vi "DMSO_load_sample_BM.vi"(6 "COM Port":refnum<visa-resource-name>="COM9", 7 "Pump Parameters":T1={"Speed 1"="100", "Speed 2"="250", "Speed 3"="250", "Speed 4"="250", "UW/Sample"="5", "Sparge"="2", "Std"="4", "Waste"="15", "Air"="14", "Milli-Q"="1", "H2SO4"="6", "NaOH"="3", "Catalyst"="7", "Cell (H+ side)"="8", "Cell (sample side)"="9", "NaCl"="9"}, 9 "step to ml":dbl=1920.0, 10 "Total Vol. (mL)":dbl, 11 "Sample Vol. (mL)":dbl=10.0) -> ()   [LabVIEW 2021]
panel:
  out "Full Command":string="o4A0V5000o1P14400o4D14400o1P33600o4D9600o2D24000o5P9600o2D9600o6P33600o4D33600"
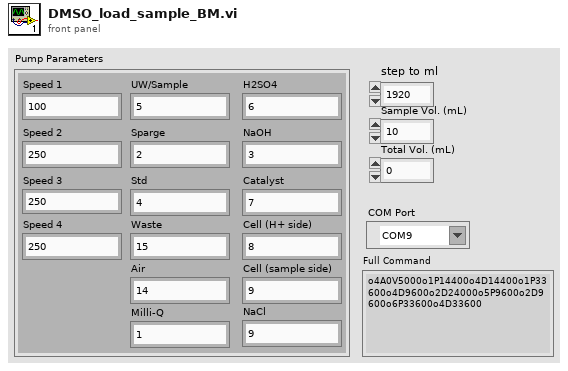
[diagram p1: front panel]
types:
  T1 = cluster{"Speed 1":string, "Speed 2":string, "Speed 3":string, "Speed 4":string, "UW/Sample":string, "Sparge":string, "Std":string, "Waste":string, "Air":string, "Milli-Q":string, "H2SO4":string, "NaOH":string, "Catalyst":string, "Cell (H+ side)":string, "Cell (sample side)":string, "NaCl":string}
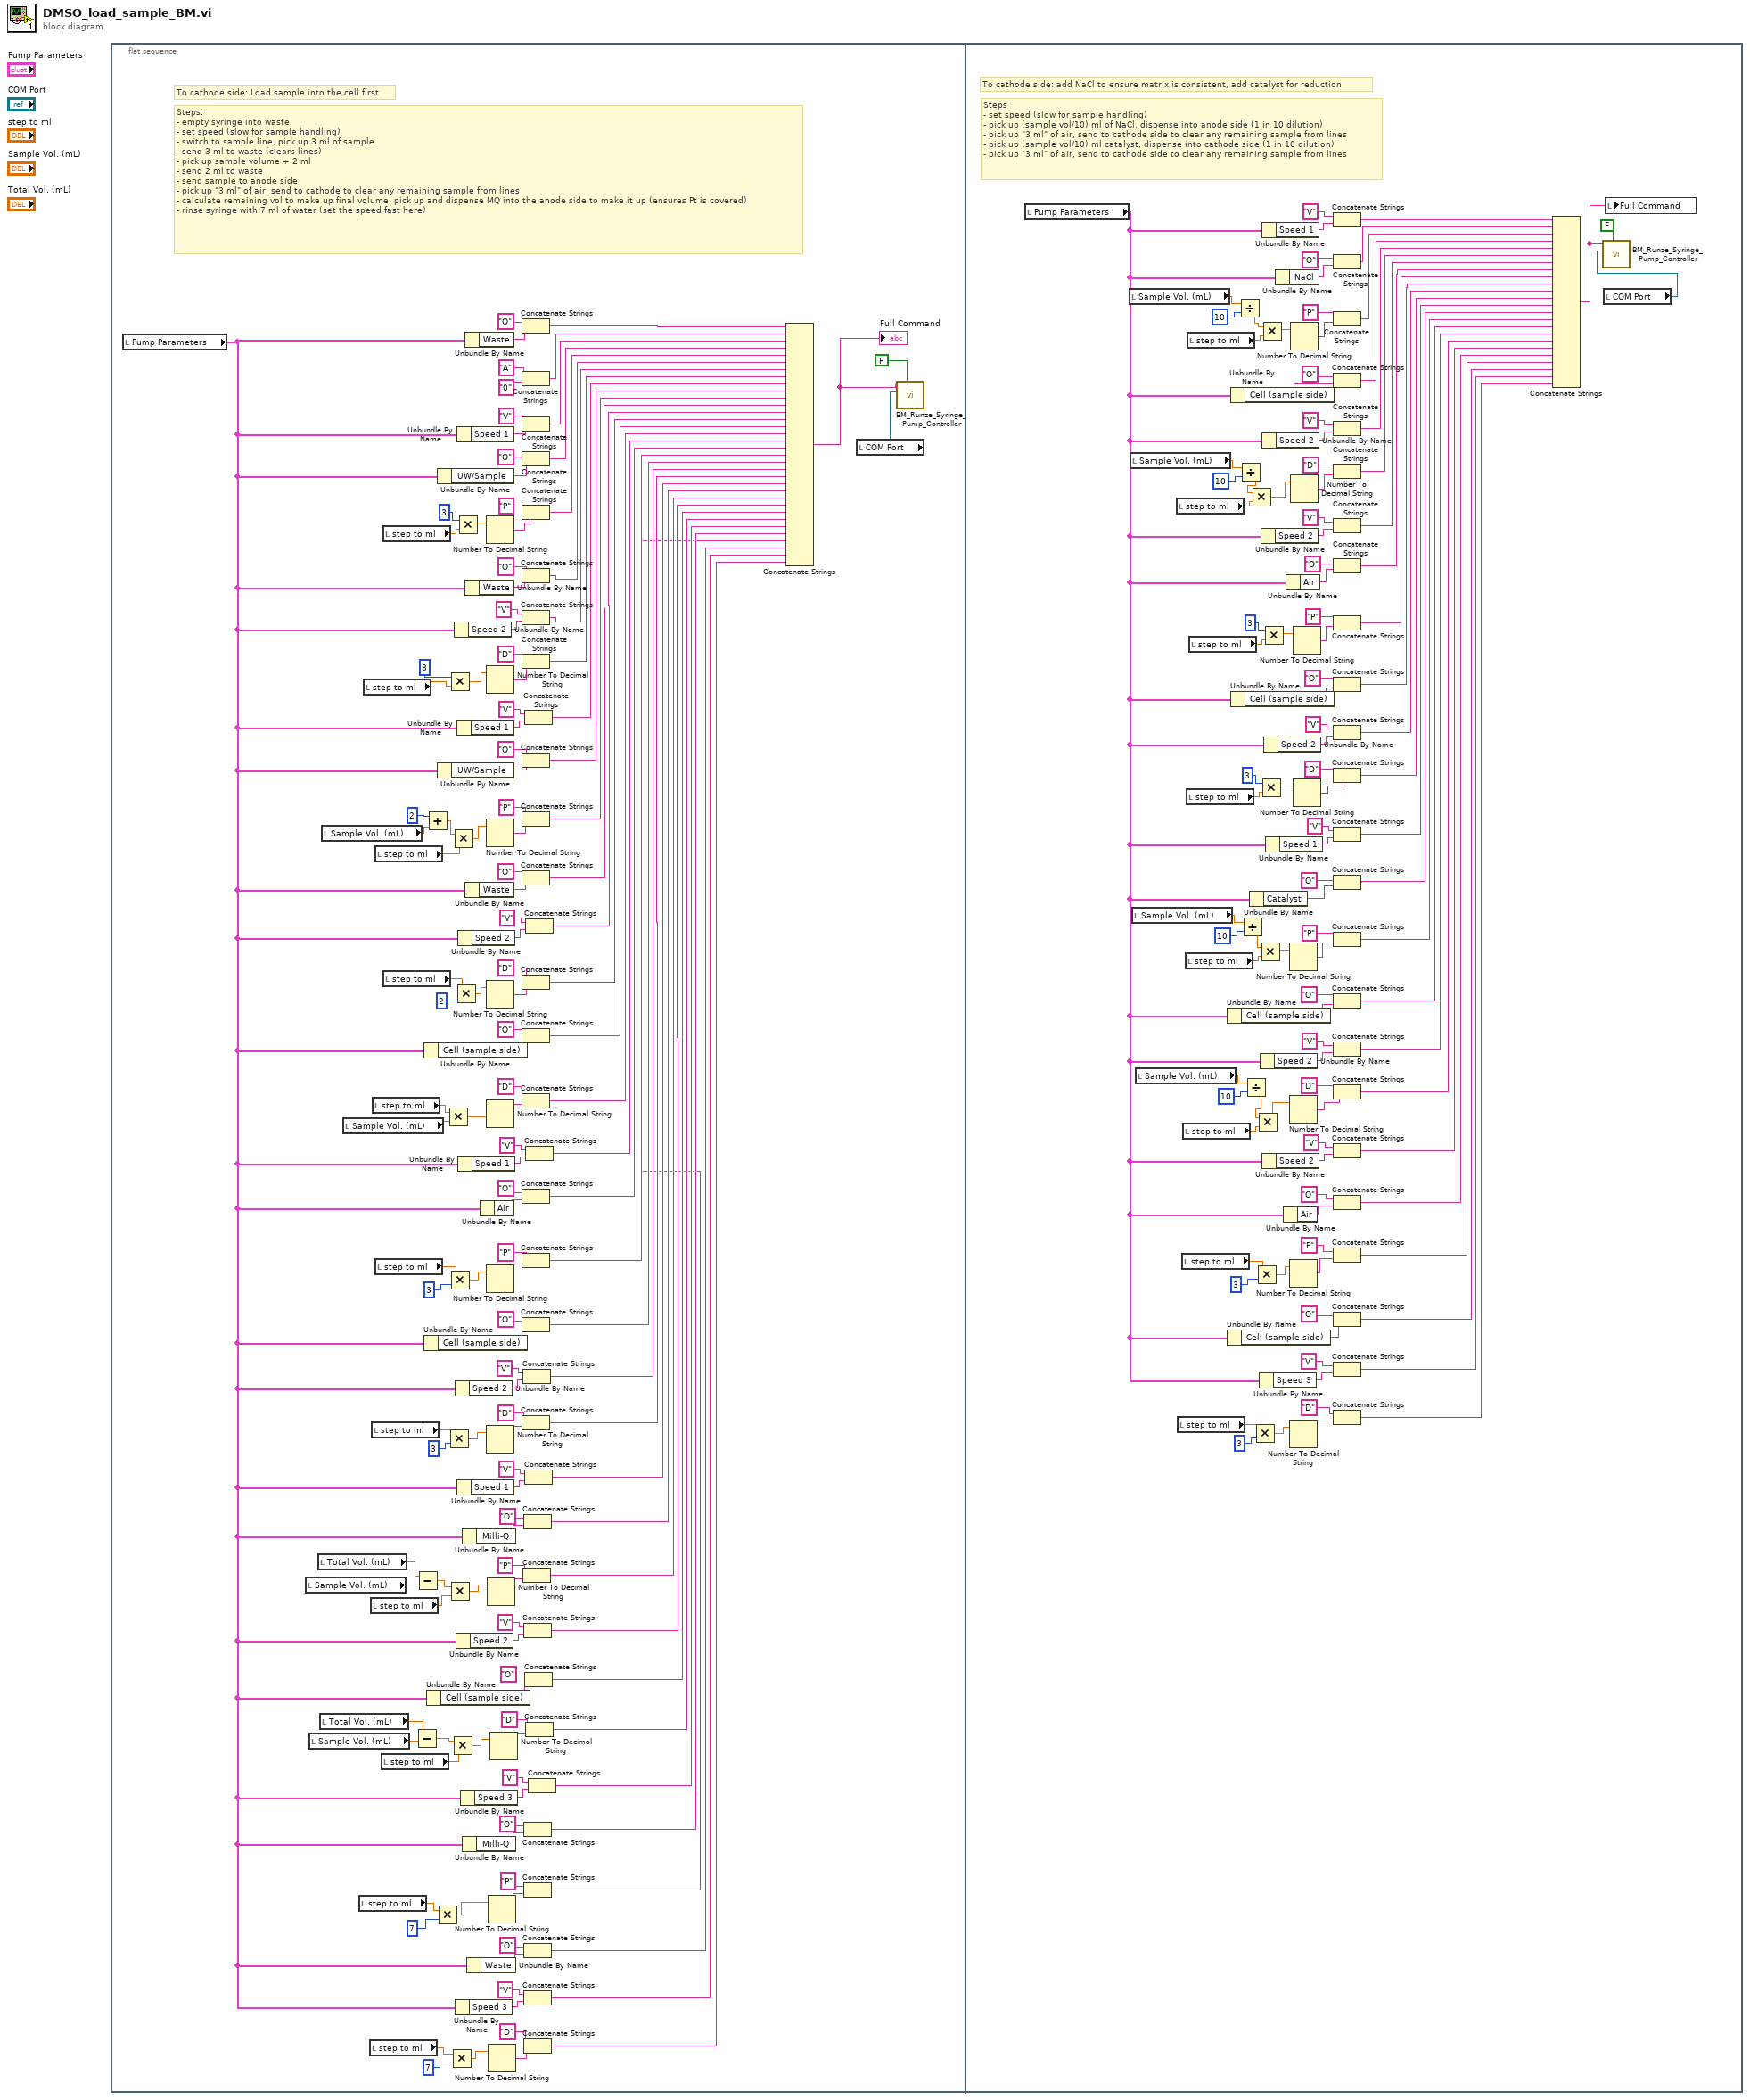
[diagram p0: block diagram]
diagram:
  n1 = flat-sequence {
    frame #0 {
      # "Steps:\n- empty syringe into waste\n- set speed (slow for sample handling)\n- switch to sample line, pick up 3 ml of sample\n- send 3 ml to waste (clears lines)\n- pick up sample volume + 2 ml\n- send 2 ml to waste\n- send sample to anode side\n- pick up \"3 ml\" of air, send to cathode to clear any remaining sample from lines\n- calculate remaining vol to make up final volume; pick up and dispense MQ into the anode side to make it up (ensures Pt is covered)\n- rinse syringe with 7 ml of water (set the speed fast here)"
      # "To cathode side: Load sample into the cell first"
      n2 = local read "Pump Parameters"() -> (w3:T1)
      n3 = local read "Sample Vol. (mL)"() -> (w2:dbl)
      n4 = local read "Sample Vol. (mL)"() -> (w1:dbl)
      n5 = local read "Total Vol. (mL)"() -> (w23:dbl)
      n6 = local read "Total Vol. (mL)"() -> (w22:dbl)
      n7 = local read "Sample Vol. (mL)"() -> (w103:dbl)
      n8 = local read "Sample Vol. (mL)"() -> (w102:dbl)
      n9 = local read "step to ml"() -> (w115:dbl)
      n10 = local read "step to ml"() -> (w97:dbl)
      n11 = local read "step to ml"() -> (w77:dbl)
      n12 = local read "step to ml"() -> (w29:dbl)
      n13 = local read "step to ml"() -> (w86:dbl)
      n14 = local read "step to ml"() -> (w117:dbl)
      n15 = local read "step to ml"() -> (w118:dbl)
      n16 = local read "step to ml"() -> (w116:dbl)
      n17 = local read "step to ml"() -> (w20:dbl)
      n18 = local read "step to ml"() -> (w120:dbl)
      n19 = local read "step to ml"() -> (w119:dbl)
      n20 = Subtract(x=w22, y=w1) -> (x-y=w21:dbl)
      n21 = Subtract(x=w23, y=w2) -> (x-y=w30:dbl)
      n22 = Add(x=2, y=w103) -> (x+y=w138:dbl)
      n23 = Unbundle By Name(w3) -> ("Cell (sample side)"=w108:string)
      n24 = Unbundle By Name(w3) -> ("Cell (sample side)"=w106:string)
      n25 = Unbundle By Name(w3) -> ("Cell (sample side)"=w27:string)
      n26 = Multiply(x=w115, y=7) -> (x*y=w135:dbl)
      n27 = Unbundle By Name(w3) -> ("UW/Sample"=w112:string)
      n28 = Unbundle By Name(w3) -> ("UW/Sample"=w110:string)
      n29 = Multiply(x=w117, y=w102) -> (x*y=w142:dbl)
      n30 = Multiply(x=w86, y=3) -> (x*y=w87:dbl)
      n31 = Multiply(x=3, y=w97) -> (x*y=w98:dbl)
      n32 = Multiply(x=w116, y=3) -> (x*y=w141:dbl)
      n33 = Multiply(x=w30, y=w29) -> (x*y=w33:dbl)
      n34 = Multiply(x=w77, y=7) -> (x*y=w79:dbl)
      n35 = Multiply(x=w21, y=w20) -> (x*y=w26:dbl)
      n36 = Multiply(x=w138, y=w118) -> (x*y=w139:dbl)
      n37 = Multiply(x=w119, y=2) -> (x*y=w144:dbl)
      n38 = Multiply(x=3, y=w120) -> (x*y=w136:dbl)
      n39 = Unbundle By Name(w3) -> ("Speed 2"=w72:string)
      n40 = Unbundle By Name(w3) -> ("Speed 2"=w64:string)
      n41 = Unbundle By Name(w3) -> ("Speed 3"=w15:string)
      n42 = Unbundle By Name(w3) -> ("Speed 2"=w18:string)
      n43 = Unbundle By Name(w3) -> ("Speed 1"=w113:string)
      n44 = Unbundle By Name(w3) -> ("Speed 1"=w71:string)
      n45 = Unbundle By Name(w3) -> ("Speed 1"=w63:string)
      n46 = Unbundle By Name(w3) -> ("Speed 2"=w68:string)
      n47 = Unbundle By Name(w3) -> ("Speed 1"=w67:string)
      n48 = Unbundle By Name(w3) -> ("Speed 3"=w17:string)
      n49 = Unbundle By Name(w3) -> ("Milli-Q"=w34:string)
      n50 = Unbundle By Name(w3) -> ("Milli-Q"=w105:string)
      n51 = Unbundle By Name(w3) -> ("Waste"=w114:string)
      n52 = Unbundle By Name(w3) -> ("Waste"=w111:string)
      n53 = Unbundle By Name(w3) -> ("Waste"=w109:string)
      n54 = Unbundle By Name(w3) -> ("Waste"=w104:string)
      n55 = Unbundle By Name(w3) -> ("Air"=w107:string)
      n56 = Number To Decimal String(number=w136) -> (decimal integer string=w96:string)  [unwired: 1 out]
      n57 = Number To Decimal String(number=w98) -> (decimal integer string=w95:string)  [unwired: 1 out]
      n58 = Number To Decimal String(number=w139) -> (decimal integer string=w93:string)  [unwired: 1 out]
      n59 = Number To Decimal String(number=w144) -> (decimal integer string=w92:string)  [unwired: 1 out]
      n60 = Number To Decimal String(number=w142) -> (decimal integer string=w89:string)  [unwired: 1 out]
      n61 = Number To Decimal String(number=w141) -> (decimal integer string=w84:string)  [unwired: 1 out]
      n62 = Number To Decimal String(number=w87) -> (decimal integer string=w82:string)  [unwired: 1 out]
      n63 = Number To Decimal String(number=w33) -> (decimal integer string=w31:string)  [unwired: 1 out]
      n64 = Number To Decimal String(number=w135) -> (decimal integer string=w80:string)  [unwired: 1 out]
      n65 = Number To Decimal String(number=w79) -> (decimal integer string=w76:string)  [unwired: 1 out]
      n66 = Number To Decimal String(number=w26) -> (decimal integer string=w24:string)  [unwired: 1 out]
      n67 = Concatenate Strings("O", w114) -> (w59:string)
      n68 = Concatenate Strings("A", "0") -> (w58:string)
      n69 = Concatenate Strings("V", w113) -> (w57:string)
      n70 = Concatenate Strings("O", w112) -> (w56:string)
      n71 = Concatenate Strings("P", w96) -> (w55:string)
      n72 = Concatenate Strings("O", w111) -> (w54:string)
      n73 = Concatenate Strings("V", w72) -> (w53:string)
      n74 = Concatenate Strings("D", w95) -> (w52:string)
      n75 = Concatenate Strings("O", w110) -> (w50:string)
      n76 = Concatenate Strings("P", w93) -> (w49:string)
      n77 = Concatenate Strings("O", w109) -> (w48:string)
      n78 = Concatenate Strings("D", w92) -> (w46:string)
      n79 = Concatenate Strings("O", w108) -> (w45:string)
      n80 = Concatenate Strings("D", w89) -> (w44:string)
      n81 = Concatenate Strings("O", w107) -> (w42:string)
      n82 = Concatenate Strings("P", w84) -> (w41:string)
      n83 = Concatenate Strings("O", w106) -> (w40:string)
      n84 = Concatenate Strings("D", w82) -> (w38:string)
      n85 = Concatenate Strings("V", w64) -> (w39:string)
      n86 = Concatenate Strings("P", w31) -> (w13:string)
      n87 = Concatenate Strings("O", w34) -> (w14:string)
      n88 = Concatenate Strings("V", w18) -> (w12:string)
      n89 = Concatenate Strings("O", w105) -> (w8:string)
      n90 = Concatenate Strings("P", w80) -> (w7:string)
      n91 = Concatenate Strings("O", w104) -> (w6:string)
      n92 = Concatenate Strings("V", w15) -> (w5:string)
      n93 = Concatenate Strings("D", w76) -> (w4:string)
      n94 = Concatenate Strings("V", w71) -> (w51:string)
      n95 = Concatenate Strings("V", w63) -> (w37:string)
      n96 = Concatenate Strings("O", w27) -> (w11:string)
      n97 = Concatenate Strings("V", w68) -> (w47:string)
      n98 = Concatenate Strings("V", w67) -> (w43:string)
      n99 = Concatenate Strings("D", w24) -> (w10:string)
      n100 = Concatenate Strings("V", w17) -> (w9:string)
      n101 = Concatenate Strings(w59, w58, w57, w56, w55, w54, w53, w52, w51, w50, w49, w48, w47, w46, w45, w44, w43, w42, w41, w40, w39, w38, w37, w14, w13, w12, w11, w10, w9, w8, w7, w6, w5, w4) -> (w123:string)
      "Full Command" <- w123
      n102 = local read "COM Port"() -> (w122:refnum<visa-resource-name>)
      n103 = call "BM_Runze_Syringe_Pump_Controller.vi"("Initialize Plunger?"=FALSE ("Initialize?"), "COM Port (Runze)"=w122, "Enter Command"=w123) -> ()  [unwired: 6 in, 3 out]
    }
    frame #1 {
      # "Steps\n- set speed (slow for sample handling)\n- pick up (sample vol/10) ml of NaCl, dispense into anode side (1 in 10 dilution)\n- pick up \"3 ml\" of air, send to cathode side to clear any remaining sample from lines\n- pick up (sample vol/10) ml catalyst, dispense into cathode side (1 in 10 dilution)\n- pick up \"3 ml\" of air, send to cathode side to clear any remaining sample from lines"
      # "To cathode side: add NaCl to ensure matrix is consistent, add catalyst for reduction"
      n104 = local read "Pump Parameters"() -> (w158:T1)
      n105 = local read "Sample Vol. (mL)"() -> (w157:dbl)
      n106 = local read "Sample Vol. (mL)"() -> (w153:dbl)
      n107 = local read "Sample Vol. (mL)"() -> (w151:dbl)
      n108 = local read "Sample Vol. (mL)"() -> (w148:dbl)
      n109 = local read "step to ml"() -> (w210:dbl)
      n110 = local read "step to ml"() -> (w230:dbl)
      n111 = local read "step to ml"() -> (w235:dbl)
      n112 = local read "step to ml"() -> (w243:dbl)
      n113 = local read "step to ml"() -> (w249:dbl)
      n114 = local read "step to ml"() -> (w186:dbl)
      n115 = local read "step to ml"() -> (w216:dbl)
      n116 = local read "step to ml"() -> (w193:dbl)
      n117 = Unbundle By Name(w158) -> ("Cell (sample side)"=w245:string)
      n118 = Unbundle By Name(w158) -> ("Cell (sample side)"=w234:string)
      n119 = Unbundle By Name(w158) -> ("Cell (sample side)"=w212:string)
      n120 = Unbundle By Name(w158) -> ("Cell (sample side)"=w189:string)
      n121 = Divide(x=w157, y=10) -> (x/y=w155:dbl)
      n122 = Divide(x=w153, y=10) -> (x/y=w152:dbl)
      n123 = Divide(x=w151, y=10) -> (x/y=w147:dbl)
      n124 = Divide(x=w148, y=10) -> (x/y=w146:dbl)
      n125 = Multiply(x=w152, y=w210) -> (x*y=w211:dbl)
      n126 = Unbundle By Name(w158) -> ("Catalyst"=w226:string)
      n127 = Multiply(x=w230, y=3) -> (x*y=w231:dbl)
      n128 = Multiply(x=w235, y=3) -> (x*y=w238:dbl)
      n129 = Multiply(x=w146, y=w243) -> (x*y=w244:dbl)
      n130 = Multiply(x=w147, y=w249) -> (x*y=w250:dbl)
      n131 = Multiply(x=3, y=w186) -> (x*y=w187:dbl)
      n132 = Multiply(x=w155, y=w216) -> (x*y=w217:dbl)
      n133 = Unbundle By Name(w158) -> ("Speed 3"=w159:string)
      n134 = Multiply(x=3, y=w193) -> (x*y=w194:dbl)
      n135 = Unbundle By Name(w158) -> ("Speed 2"=w222:string)
      n136 = Unbundle By Name(w158) -> ("Speed 2"=w178:string)
      n137 = Unbundle By Name(w158) -> ("Speed 1"=w251:string)
      n138 = Unbundle By Name(w158) -> ("Speed 2"=w206:string)
      n139 = Unbundle By Name(w158) -> ("Speed 2"=w177:string)
      n140 = Unbundle By Name(w158) -> ("Speed 2"=w182:string)
      n141 = Unbundle By Name(w158) -> ("Speed 1"=w180:string)
      n142 = Unbundle By Name(w158) -> ("NaCl"=w204:string)
      n143 = Unbundle By Name(w158) -> ("Air"=w239:string)
      n144 = Unbundle By Name(w158) -> ("Air"=w179:string)
      n145 = Number To Decimal String(number=w250) -> (decimal integer string=w247:string)  [unwired: 1 out]
      n146 = Number To Decimal String(number=w244) -> (decimal integer string=w241:string)  [unwired: 1 out]
      n147 = Number To Decimal String(number=w238) -> (decimal integer string=w232:string)  [unwired: 1 out]
      n148 = Number To Decimal String(number=w231) -> (decimal integer string=w227:string)  [unwired: 1 out]
      n149 = Number To Decimal String(number=w217) -> (decimal integer string=w214:string)  [unwired: 1 out]
      n150 = Number To Decimal String(number=w211) -> (decimal integer string=w208:string)  [unwired: 1 out]
      n151 = Number To Decimal String(number=w194) -> (decimal integer string=w191:string)  [unwired: 1 out]
      n152 = Number To Decimal String(number=w187) -> (decimal integer string=w184:string)  [unwired: 1 out]
      n153 = Concatenate Strings("V", w251) -> (w203:string)
      n154 = Concatenate Strings("O", w204) -> (w202:string)
      n155 = Concatenate Strings("P", w214) -> (w201:string)
      n156 = Concatenate Strings("O", w212) -> (w200:string)
      n157 = Concatenate Strings("V", w206) -> (w199:string)
      n158 = Concatenate Strings("D", w208) -> (w198:string)
      n159 = Concatenate Strings("V", w178) -> (w197:string)
      n160 = Concatenate Strings("O", w179) -> (w176:string)
      n161 = Concatenate Strings("P", w191) -> (w175:string)
      n162 = Concatenate Strings("O", w189) -> (w174:string)
      n163 = Concatenate Strings("V", w182) -> (w173:string)
      n164 = Concatenate Strings("D", w184) -> (w172:string)
      n165 = Concatenate Strings("V", w180) -> (w171:string)
      n166 = Concatenate Strings("O", w226) -> (w170:string)
      n167 = Concatenate Strings("P", w247) -> (w169:string)
      n168 = Concatenate Strings("O", w245) -> (w168:string)
      n169 = Concatenate Strings("V", w222) -> (w167:string)
      n170 = Concatenate Strings("D", w241) -> (w166:string)
      n171 = Concatenate Strings("V", w177) -> (w165:string)
      n172 = Concatenate Strings("O", w239) -> (w164:string)
      n173 = Concatenate Strings("P", w232) -> (w163:string)
      n174 = Concatenate Strings("O", w234) -> (w162:string)
      n175 = Concatenate Strings("V", w159) -> (w161:string)
      n176 = Concatenate Strings("D", w227) -> (w160:string)
      n177 = Concatenate Strings(w203, w202, w201, w200, w199, w198, w197, w176, w175, w174, w173, w172, w171, w170, w169, w168, w167, w166, w165, w164, w163, w162, w161, w160) -> (w224:string)
      n178 = local read "COM Port"() -> (w225:refnum<visa-resource-name>)
      n179 = call "BM_Runze_Syringe_Pump_Controller.vi"("Initialize Plunger?"=FALSE ("Initialize?"), "COM Port (Runze)"=w225, "Enter Command"=w224) -> ()  [unwired: 6 in, 3 out]
      n180 = local write "Full Command"(w224) -> ()
    }
  }
